vi "CCM-Read Connection Tables (by device).vi"(0 "Path In":path, 7 "Channels By Device":cluster{"Out":string[], "In":string[]}[](array[cluster]), 11 "error in (no error)":errorcluster) -> (4 "Path Out":path, 6 "Tables By Device":T1(array[cluster]), 15 "error out":errorcluster)   [LabVIEW 2020]
uses:
  Type Defs/CM-IO Type.ctl
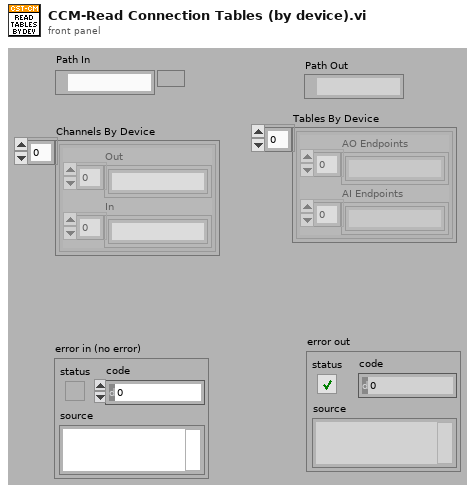
[diagram p1: front panel]
types:
  T1 = cluster{"AO Endpoints":string[], "AI Endpoints":string[]}[]
  T2 = typedef "CM-IO Type.ctl" = enum16{"Analog Outputs", "Analog Inputs", "Digital Outputs", "Digital Inputs"}
  T3 = cluster{"Endpoints (by channel)":string[], "Endpoints (by channel)":string[]}
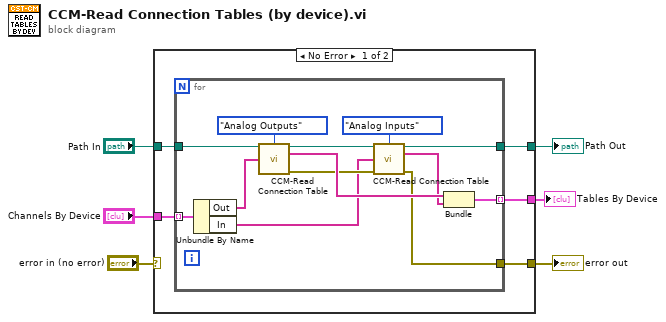
[diagram p0: block diagram]
diagram:
  n1 = case shown="No Error" "error in (no error)" {
    selector: "error in (no error)" -> [_ w26]
    tunnel: "Channels By Device" -> [w11 _]
    tunnel: "Path In" -> [w10 w25]
    tunnel: [w8 w26] -> w3
    tunnel: [w9 w25] -> w2
    tunnel: [w7 _] -> w1
    frame No Error {
      n2 = for {
        tunnel: w11 -> [w24] mode=indexing
        tunnel: w10 -> [w22]
        tunnel: [w15] -> w9
        tunnel: [w20] -> w7 mode=indexing
        tunnel: [w13] -> w8
        n3 = Unbundle By Name(w24) -> ("Out"=w23:string[], "In"=w14:string[])
        n4 = call "CCM-Read Connection Table.vi"("Path In"=w22, "Type"=CM-IO_Type."Analog Outputs", "IOChannels"=w23) -> ("Path Out"=w17:path, "Endpoints (by channel)"=w21:string[], "error out"=w16:errorcluster)  [unwired: 9 in, 1 out]
        n5 = call "CCM-Read Connection Table.vi"("Path In"=w17, "Type"=CM-IO_Type."Analog Inputs", "IOChannels"=w14, "error in (no error)"=w16) -> ("Path Out"=w15:path, "Endpoints (by channel)"=w12:string[], "error out"=w13:errorcluster)  [unwired: 8 in, 1 out]
        n6 = Bundle("Endpoints (by channel)"=w21, "Endpoints (by channel)"=w12) -> (w20:T3)  [unwired: 1 in]
      }
    }
    frame Error {
    }
  }
  "error out" <- w3
  "Path Out" <- w2
  "Tables By Device" <- w1
